vi "Pack Multiple 24xI16 to 32xI16_debug.vi"(8 "Input Valid":bool, 11 "Input Data":i16[](array[numeric])=[0, 0, 0, 0, 0, 0, 0, 0, 0, 0, 0, 0, 0, 0, 0, 0, 0, 0, 0, 0, 0, 0, 0, 0]) -> (0 "Output Valid":bool, 3 "Output Data":i16[](array[numeric]))   [LabVIEW 2012]
doc: "<b> Latency = 2 Ticks </b>"
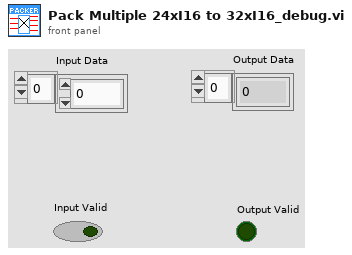
[diagram p1: front panel]
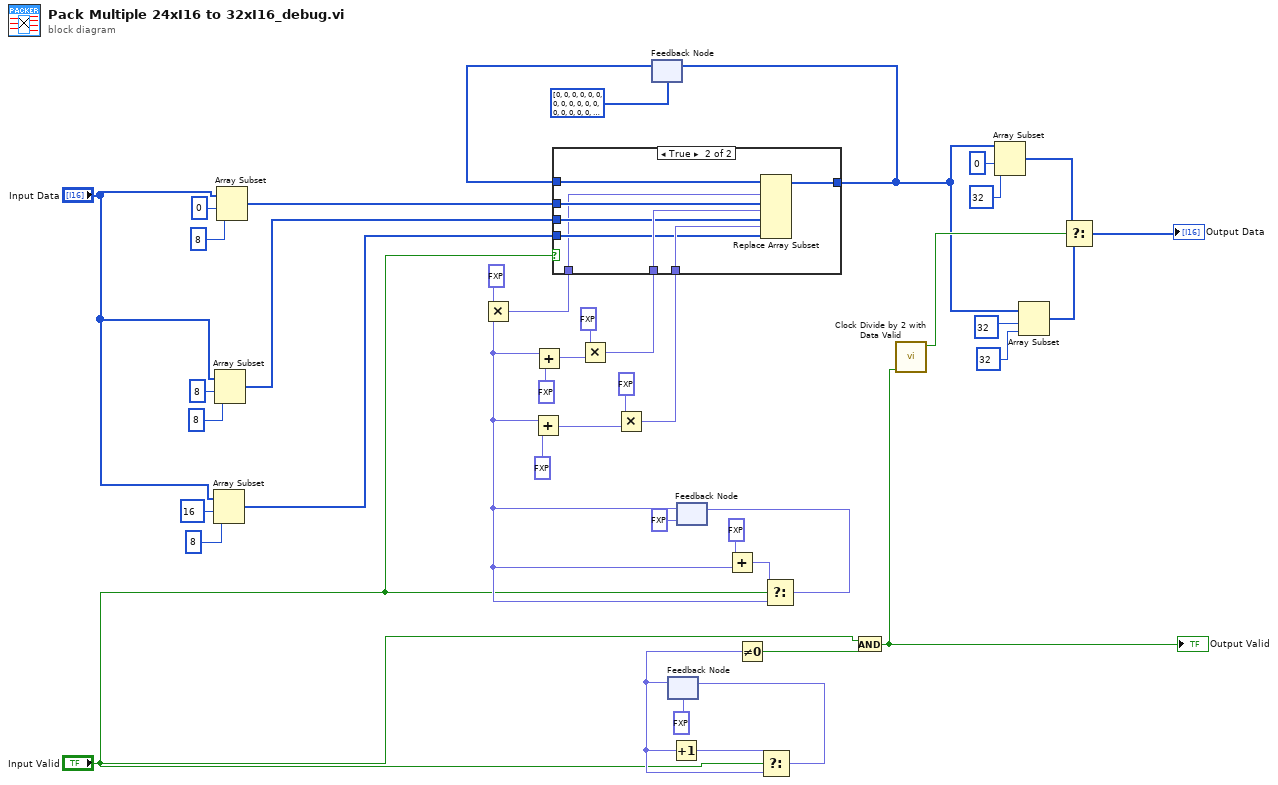
[diagram p0: block diagram]
diagram:
  n1 = Array Subset(array="Input Data", index=16, length=8) -> (w21:i16[])
  n2 = Array Subset(array="Input Data", index=8, length=8) -> (w24:i16[])
  n3 = Array Subset(array="Input Data", index=0, length=8) -> (w29:i16[])
  n4 = feedback #1(i16[] [0, 0, 0, 0, 0, 0, 0, 0, 0, 0, 0, 0, 0, 0, 0, 0, 0, 0, 0, 0, 0, 0, 0, 0, 0, 0, 0, 0, 0, 0, 0, 0, 0, 0, 0, 0, 0, 0, 0, 0, 0, 0, 0, 0, 0, 0, 0, 0, 0, 0, 0, 0, 0, 0, 0, 0, 0, 0, 0, 0, 0, 0, 0, 0]) -> (w42:i16[])
  n5 = feedback #2(fxp<+,2,2> 0.0) -> (w34:fxp<+,2,2>)
  n6 = Increment(x=w34) -> (x+1=w35:fxp<+,2,2>)
  n7 = feedback #3(fxp<+,3,3> 0.0) -> (w31:fxp<+,3,3>)
  n8 = Multiply(x=fxp<+,4,4> 8.0, y=w31) -> (x*y=w19:fxp<+,7,7>)
  n9 = Add(x=w31, y=fxp<+,3,3> 2.0) -> (x+y=w15:fxp<+,3,3>)
  n10 = Add(x=w31, y=fxp<+,3,3> 1.0) -> (x+y=w18:fxp<+,3,3>)
  n11 = Multiply(x=fxp<+,4,4> 8.0, y=w18) -> (x*y=w16:fxp<+,7,7>)
  n12 = Multiply(x=fxp<+,4,4> 8.0, y=w15) -> (x*y=w14:fxp<+,7,7>)
  n13 = case shown="True" "Input Valid" {
    tunnel: w42 -> [w44 w52]
    tunnel: w16 -> [_ w51]
    tunnel: w14 -> [_ w50]
    tunnel: [w44 w49] -> w2
    tunnel: w29 -> [_ w48]
    tunnel: w24 -> [_ w47]
    tunnel: w21 -> [_ w46]
    tunnel: w19 -> [_ w45]
    frame False {
    }
    frame True {
      n14 = Replace Array Subset(array=w52, new element #1=w48, index #1=w45, new element #2=w47, index #2=w51, new element #3=w46, index #3=w50) -> (w49:i16[])
    }
  }
  n15 = feedback-in #1(w2) -> ()
  n16 = Add(x=fxp<+,3,3> 3.0, y=w31) -> (x+y=w32:fxp<+,3,3>)
  n17 = Not Equal To 0?(x=w34) -> (x != 0?=w33:bool)
  n18 = Select(t=w35, s="Input Valid", f=w34) -> (s? t:f=w36:fxp<+,2,2>)
  n19 = feedback-in #2(w36) -> ()
  n20 = Select(t=w32, s="Input Valid", f=w31) -> (s? t:f=w11:fxp<+,3,3>)
  n21 = feedback-in #3(w11) -> ()
  n22 = And(x="Input Valid", y=w33) -> (x .and. y?=w9:bool)
  "Output Valid" <- w9
  n23 = call <userlib>:"Clock Divide by 2 with Data Valid.vi"("Data Valid"=w9) -> ("CLK/2"=w10:bool)  [unwired: 10 in]
  n24 = Array Subset(array=w2, index=0, length=32) -> (w4:i16[])
  n25 = Array Subset(array=w2, index=32, length=32) -> (w3:i16[])
  n26 = Select(t=w4, s=w10, f=w3) -> (s? t:f=→"Output Data":i16[])
